vi "NeedRecalcPath.vi"(4 "SmoothPath":dbl[][](array[numeric]), 5 "Initial State":dbl[](array[numeric]), 7 "Pos x,y":dbl[](array[numeric]), 9 "IA State":T1={"our_robots"=[], "enemy_robots"=[], "balls"=[], "geometry"={"field_length"=0, "field_width"=0, "goal_width"=0, "goal_depth"=0, "center_circle_radius"=0, "defense_width"=0, "defense_depth"=0, "free_kick_from_defense_dist"=0, "penalty_spot_from_field_line_dist"=0, "penalty_line_from_spot_dist"=0, "half_moon_depth"=0, "half_moon_width"=0}, "IA Judge"={"stage"="", "command"="", "our_goalie_id"=0.0, "enemy_goalie_id"=0.0, "command enum"=enum."Halt", "Time"=enum."Azul"}, "Received Timestamp"=timestamp(0 s since 1904-01-01), "Events"={"Touch"=FALSE, "id touch"=0.0, "Ball out of \nVision"=FALSE, "Ball inside \nGoalie area"=FALSE, "Robot not responding"=FALSE, "Robots responding status"=[1.0, 1.0, 1.0, 1.0, 1.0, 1.0], "Enemy Ball \nPossession"=FALSE, "Id ini Possession"=0.0, "Ball Possesion"=FALSE, "Id Possesion"=0.0, "Ball at\nour goal side"=FALSE, "Ball at\ntouchline"=FALSE, "Ball at\nenemy goal side"=FALSE}}, 10 "Robot":T2, 11 "Dest x,y":dbl[](array[numeric])) -> (3 "Boolean":bool)   [LabVIEW 2018]
uses:
  Core/AI Robot.ctl
  Intel/Functions Enum.ctl
  Intel/AttackerStates.ctl
  PathDests.ctl
  PathDest.ctl
  Core/AI Input.ctl
  Core/AI Ball.ctl
  Core/Field Size.ctl
  Core/AI Judge.ctl
  Intel/Command Enum.ctl
  Util/Events/Events.ctl
  <vilib>/Analysis/_algsub.llb/Real Vector Norm.vi
  <vilib>/Analysis/NI_AALPro.lvlib
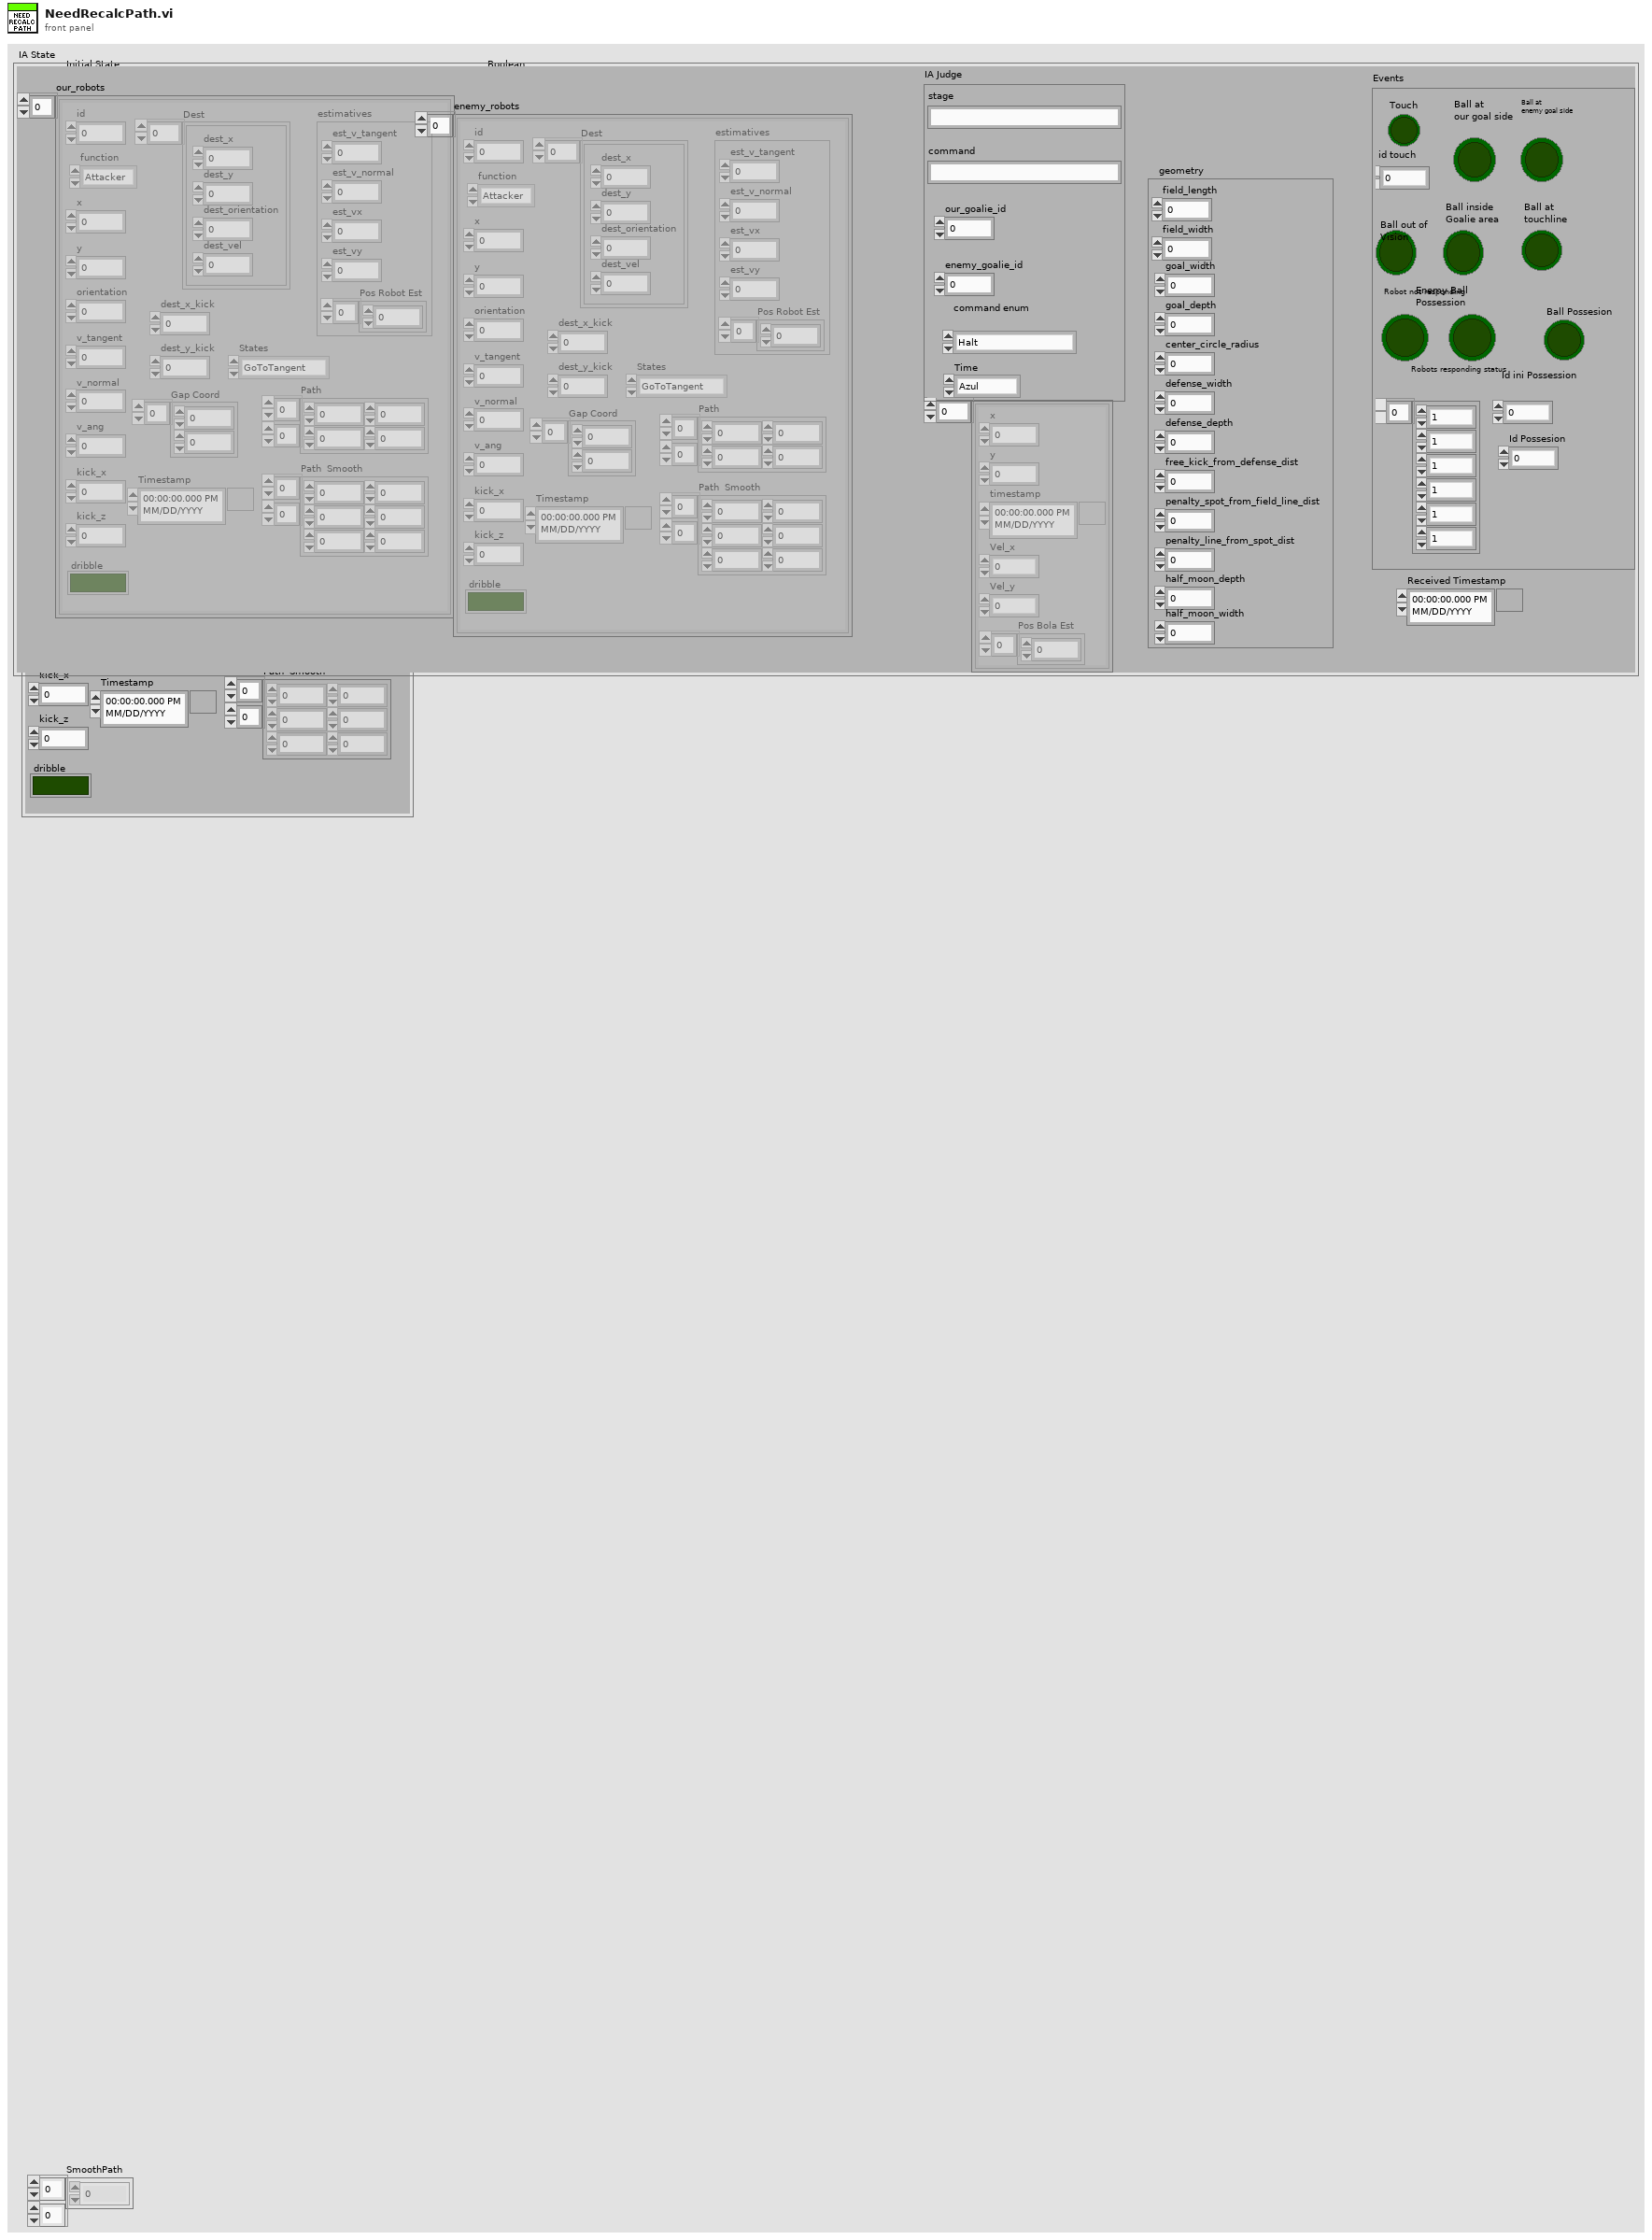
[diagram p1: front panel]
types:
  T1 = typedef "AI Input.ctl" = cluster{"our_robots":T2[], "enemy_robots":T2[], "balls":T7[], "geometry":T8, "IA Judge":T9, "Received Timestamp":timestamp, "Events":T11}
  T2 = typedef "AI Robot.ctl" = cluster{"id":u32, "function":T3, "x":dbl, "y":dbl, "orientation":dbl, "v_tangent":dbl, "v_normal":dbl, "v_ang":dbl, "kick_x":dbl, "kick_z":dbl, "dribble":bool, "Timestamp":timestamp, "estimatives":cluster{"est_v_tangent":dbl, "est_v_normal":dbl, "est_vx":dbl, "est_vy":dbl, "Pos Robot Est":dbl[]}, "dest_x_kick":dbl, "dest_y_kick":dbl, "Gap Coord":dbl[], "States":T4, "Path ":dbl[][], "Path  Smooth":dbl[][], "Dest":T5}
  T3 = typedef "Functions Enum.ctl" = enum16{"Attacker", "Goalie", "Defender", "Striker", "Goto 0", "Dummy", "Kicker", "ZigZag"}
  T4 = typedef "AttackerStates.ctl" = enum16{"Pass", "GoToTangent", "BallGetting", "GoToKick", "Rotate anti-clockwise", "Rotate Clockwise", ""}
  T5 = typedef "PathDests.ctl" = T6[]
  T6 = typedef "PathDest.ctl" = cluster{"dest_x":dbl, "dest_y":dbl, "dest_orientation":dbl, "dest_vel":dbl}
  T7 = typedef "AI Ball.ctl" = cluster{"x":dbl, "y":dbl, "timestamp":timestamp, "Vel_x":dbl, "Vel_y":dbl, "Pos Bola Est":dbl[]}
  T8 = typedef "Field Size.ctl" = cluster{"field_length":u32, "field_width":u32, "goal_width":u32, "goal_depth":u32, "center_circle_radius":u32, "defense_width":u32, "defense_depth":u32, "free_kick_from_defense_dist":u32, "penalty_spot_from_field_line_dist":u32, "penalty_line_from_spot_dist":u32, "half_moon_depth":u32, "half_moon_width":u32}
  T9 = typedef "AI Judge.ctl" = cluster{"stage":string, "command":string, "our_goalie_id":dbl, "enemy_goalie_id":dbl, "command enum":T10, "Time":enum16{"Azul", "Amarelo"}}
  T10 = typedef "Command Enum.ctl" = enum16{"Halt", "Stop", "Force Start", "PKA Normal Start", "Prepare Kickoff Ally", "PKE Normal Start", "Prepare Kickoff Enemy", "Prepare Penalty Ally", "PPA Normal Start", "Prepare Penalty Enemy", "PPE Normal Start", "Ball Placement Enemy Up", "Ball Placement Enemy Down", "Ball Placement Ally Up", "Ball Placement Ally Mid", "Ball Placement Ally Down", "Indirect Free Enemy", "Indirect Free Ally", "Timeout Enemy", "Timeout Ally", "Goal Enemy", "Goal Ally", "Normal Half Time", "Extra Time Break", "Extra Half Time", "None", "Post Game"}
  T11 = typedef "Events.ctl" = cluster{"Touch":bool, "id touch":dbl, "Ball out of \nVision":bool, "Ball inside \nGoalie area":bool, "Robot not responding":bool, "Robots responding status":dbl[], "Enemy Ball \nPossession":bool, "Id ini Possession":dbl, "Ball Possesion":bool, "Id Possesion":dbl, "Ball at\nour goal side":bool, "Ball at\ntouchline":bool, "Ball at\nenemy goal side":bool}
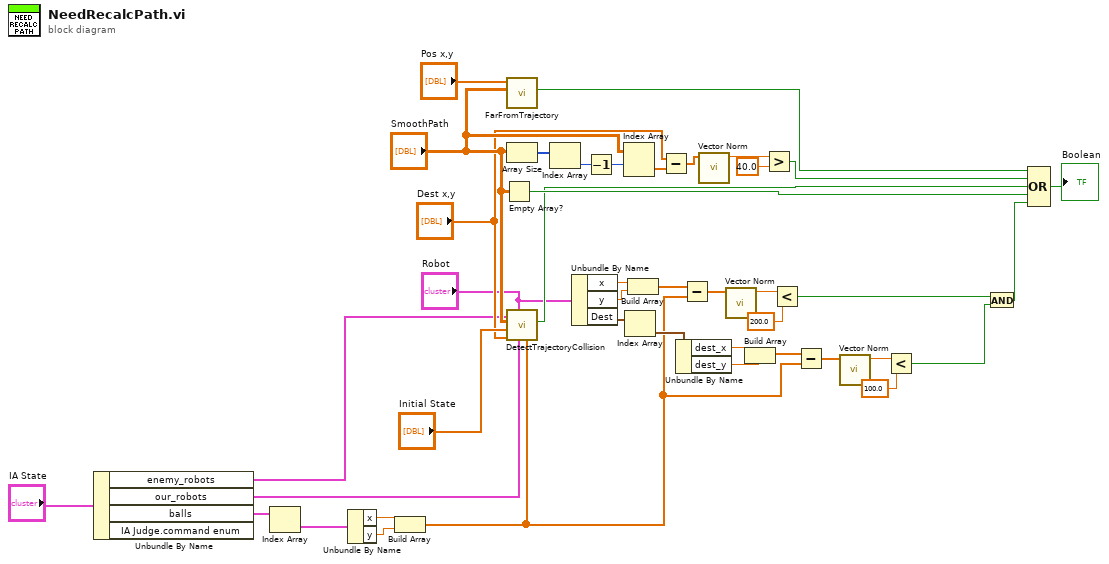
[diagram p0: block diagram]
diagram:
  n1 = Unbundle By Name("IA State") -> ("enemy_robots"=w25:T2[], "our_robots"=w24:T2[], "balls"=w23:T7[])  [unwired: 1 out]
  n2 = Index Array(array=w23) -> (element=w22:T7)  [unwired: 1 in]
  n3 = Unbundle By Name(w22) -> ("x"=w17:dbl, "y"=w16:dbl)
  n4 = Build Array(w17, w16) -> (w1:dbl[])
  n5 = Empty Array?(array="SmoothPath") -> (empty?=w37:bool)
  n6 = call "FarFromTrajectory.vi"("Path"="SmoothPath", "Position"="Pos x,y") -> ("Far from trajectory?"=w39:bool)  [unwired: 9 in]
  n7 = Array Size(array="SmoothPath") -> (size(s)=w28:i32[])
  n8 = call "DetectTrajectoryCollision.vi"("ball"=w1, "our_robots"=w24, "Robot in"="Robot", "Goal"="Dest x,y", "Initial State"="Initial State", "Last Path"="SmoothPath", "enemy_robots"=w25) -> ("Collision"=w27:bool)  [unwired: 4 in]
  n9 = Index Array(array=w28) -> (element=w35:i32)  [unwired: 1 in]
  n10 = Unbundle By Name("Robot") -> ("x"=w20:dbl, "y"=w19:dbl, "Dest"=w13:T5)
  n11 = Decrement(x=w35) -> (x-1=w34:i32)
  n12 = Index Array(array="SmoothPath", index (row)=w34) -> (element=w29:dbl[])  [unwired: 1 in]
  n13 = Index Array(array=w13) -> (element=w12:T6)  [unwired: 1 in]
  n14 = Build Array(w20, w19) -> (w18:dbl[])
  n15 = Subtract(x="Dest x,y", y=w29) -> (x-y=w30:dbl[])
  n16 = Unbundle By Name(w12) -> ("dest_x"=w10:dbl, "dest_y"=w9:dbl)
  n17 = Subtract(x=w18, y=w1) -> (x-y=w15:dbl[])
  n18 = call-poly <vilib>:"Vector Norm.vi"("Input Vector"=w30) -> ("norm"=w31:dbl)  [unwired: 9 in, 1 out]
  n19 = call-poly <vilib>:"Vector Norm.vi"("Input Vector"=w15) -> ("norm"=w14:dbl)  [unwired: 9 in, 1 out]
  n20 = Build Array(w10, w9) -> (w3:dbl[])
  n21 = Greater?(x=w31, y=40.0) -> (0:w32:bool)
  n22 = Less?(x=w14, y=200.0) -> (x < y?=w8:bool)
  n23 = Subtract(x=w3, y=w1) -> (x-y=w4:dbl[])
  n24 = call-poly <vilib>:"Vector Norm.vi"("Input Vector"=w4) -> ("norm"=w5:dbl)  [unwired: 9 in, 1 out]
  n25 = Less?(x=w5, y=100.0) -> (x < y?=w2:bool)
  n26 = And(x=w8, y=w2) -> (x .and. y?=w7:bool)
  n27 = Compound Arithmetic op=OR(w39, w32, w27, w37, w7) -> (→"Boolean":bool)
